vi "Create Filter Wrapper.vi"   [LabVIEW 2012, in "nisyscfg.lvlib"]
doc: "Creates a system filter object that is used to query for specific resources in a system. After creating a filter, set one or more properties using the Property Node (Filter) to limit the set of detected resources."
uses:
  <vilib>/nisyscfg/nisyscfg.lvlib
  <resource>/objmgr/nisysapi.rc
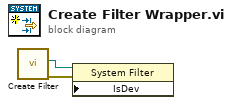
[diagram p0: block diagram]
diagram:
  n1 = call <vilib>:"Create Filter.vi"() -> ("error out"=w1:errorcluster, "Filter out"=w2:refnum<k20>)  [unwired: 9 in, 1 out]
  n2 = property class="System Filter" props=["IsDev"](reference=w2, error in=w1) -> ()  [unwired: 1 in, 2 out]
